vi "3-6.vi"() -> ()   [LabVIEW 2017]
panel:
  out "布尔":bool
  in  "数值":dbl
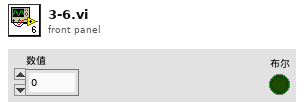
[diagram p1: front panel]
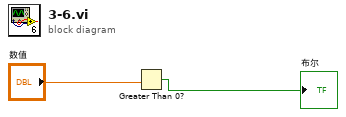
[diagram p0: block diagram]
diagram:
  n1 = Greater Than 0?(x="数值") -> (x > 0?=→"布尔":bool)
